vi "Trainning Done.vi"() -> ()   [LabVIEW 2020]
panel:
  in  "Trainning Done":bool
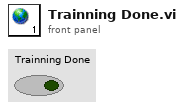
[diagram p1: front panel]
diagram:
